vi "Get Field Calibration List.vi"(7 "MCListbox 참조 번호":refnum<vi>, 8 "에러 입력":errorcluster caption="에러 입력(에러 없음)", 11 "template (empty)":path caption="템플릿(비어있음)") -> (0 "에러 출력":errorcluster, 3 "MD5 message-digest":string caption="MD5")   [LabVIEW 2020]
uses:
  <vilib>/Utility/NIReport.llb/Report Type.ctl
  <vilib>/security/Message Digest/API/Instances/File/SHA-256 File Checksum.vi
  <vilib>/addons/_office/excel.llb/Excel Get Data ([str]).vi
  Public/Polymorph/Cell Space_ListBox.vi
  <vilib>/Utility/NIReport.llb/NI_report.lvclass
  <vilib>/Utility/NIReport.llb/Excel/NI_Excel.lvclass
  <vilib>/addons/_office/NI_ReportGenerationToolkit.lvlib
  <vilib>/Utility/NIReport.llb/NI_ReportGenerationCore.lvlib
  <vilib>/security/Message Digest/API/NI_Message Digest API.lvlib
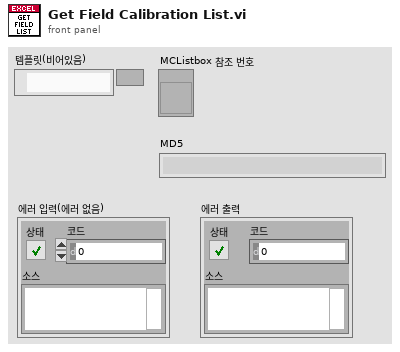
[diagram p1: front panel]
types:
  T1 = typedef "NI_ReportGenerationCore.lvlib/Report Type.ctl" = enum16{"HTML", "Word", "Excel"}
  T2 = cluster{"position (excel)":cluster{"row":i32, "column":i32}, "name (excel)":string, "bookmark (word)":string}
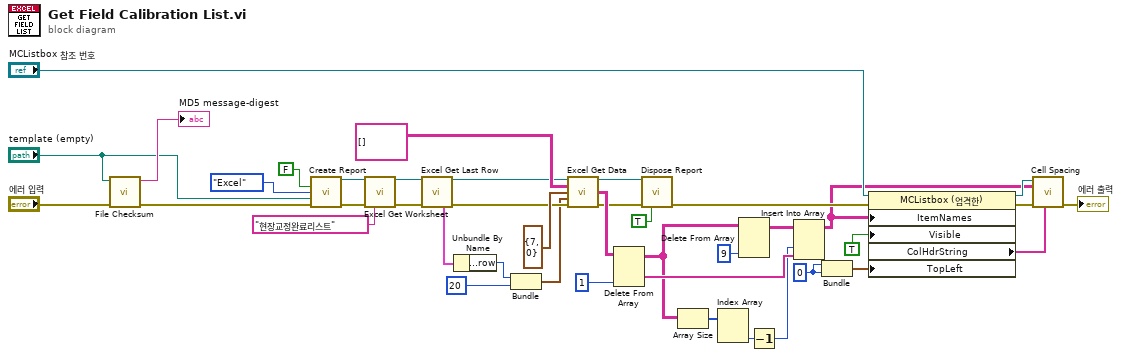
[diagram p0: block diagram]
diagram:
  w4 = 0
  n1 = call-poly <vilib>:"File Checksum.vi"("error in"="에러 입력", "path"="template (empty)") -> ("error out"=w17:errorcluster, "digest"=→"MD5 message-digest":string)  [unwired: 8 in]
  n2 = call <vilib>:"Create Report.vi"("display alerts? (F)"=FALSE, "report type"=Report_Type."Excel", "template (empty)"="template (empty)", "error in (no error)"=w17) -> ("report out"=w15:refnum<class "NI_report.lvclass">, "error out"=w16:errorcluster)  [unwired: 10 in]
  n3 = call <vilib>:"Excel Get Worksheet.vi"("report in"=w15, "error in (no error)"=w16, "name (\"\")"="현장교정완료리스트" ("name (\"\")")) -> ("report out"=w33:refnum<class "NI_report.lvclass">, "error out"=w34:errorcluster)  [unwired: 11 in]
  n4 = call <vilib>:"Excel Get Last Row.vi"("report in"=w33, "error in (no error)"=w34) -> ("report out"=w32:refnum<class "NI_report.lvclass">, "MS Office parameters out"=w31:T2)  [unwired: 11 in, 1 out]
  n5 = Unbundle By Name(w31) -> ("position (excel).row"=w30:i32)
  n6 = Bundle("row"=w30, "column"=20) -> (w28:cluster{"row":i32, "column":i32})  [unwired: 1 in]
  n7 = call-poly <vilib>:"Excel Get Data.vi"("report in"=w32, "data type"=string[][] [], "start (-1, -1)"=cluster{"row":i32, "column":i32} {"row"=7, "column"=0}, "end (-1, -1)"=w28, "error in (no error)"=w34) -> ("report out"=w40:refnum<class "NI_report.lvclass">, "data"=w25:string[][], "error out"=w20:errorcluster)  [unwired: 8 in]
  n8 = Delete From Array(array=w25, index (col)=1 ("비활성화된 인덱스 (열)")) -> (deleted portion=w26:string[], array with subset deleted=w24:string[][])  [unwired: 2 in]
  n9 = call-dynamic "Dispose Report.vi"("report in"=w40, "error in (no error)"=w20, "close report? (T)"=TRUE) -> ("error out"=w19:errorcluster)  [unwired: 12 in]
  n10 = Array Size(array=w24) -> (size(s)=w11:i32[])
  n11 = Index Array(array=w11) -> (element #2=w10:i32)  [unwired: 2 in, 1 out]
  n12 = Delete From Array(array=w24, index (col)=9 ("비활성화된 인덱스 (열)")) -> (array with subset deleted=w12:string[][])  [unwired: 2 in, 1 out]
  n13 = Decrement(x=w10) -> (x-1=w9:i32)
  n14 = Insert Into Array(array=w12, index (col)=w9, new element=w26) -> (w6:string[][])  [unwired: 1 in]
  n15 = Bundle(w4, w4) -> (w3:cluster{i32, i32})  [unwired: 1 in]
  n16 = property on="프로퍼티 노드" class="MCListbox (엄격한)"(reference="MCListbox 참조 번호", error in=w19, "ItemNames"=w6, "Visible"=TRUE ("보이기"), "TopLeft"=w3) -> (reference out=w7:refnum<vi>, error out=w8:errorcluster, "ColHdrString"=w5:string[])
  n17 = call-poly "Cell Spacing.vi"("Col Header in"=w5, "error in"=w8, "Data in"=w6, "여러열리스트박스 참조 in"=w7) -> ("error out"=→"에러 출력":errorcluster)  [unwired: 6 in, 1 out]
